vi "ProgramControl-AutoFaultRecovery.vi"(0 "Universal Robot.lvclass in":refnum<class "Universal Robot.lvclass">, 1 "Program":string, 5 "error in (no error)":errorcluster, 9 "Subpanel":refnum<vi>, 11 "Require Normal Mode to Play (F)":bool) -> (14 "Universal Robot.lvclass out":refnum<class "Universal Robot.lvclass">, 15 "programReturnStatus":T1=enum."Complete", 19 "error out":errorcluster)   [LabVIEW 2019, in "Universal Robot.lvclass"]
uses:
  Universal Robot.lvclass
  ProgramReturnStatus.ctl
  ProgramControlFPControls.ctl
  ProgramState.ctl
  SafetyStatus.ctl
  Events/Robot Event/Event Type.ctl
  Events/Robot Event/Robot Event.lvclass
panel:
  out "Loaded Program":string
  out "Message":string
  out "Program Status":string
  in  "Recover":bool
  in  "Resume":bool
  in  "auto fault timeout":i32=1000
  in  "check status timeout":i32=1000
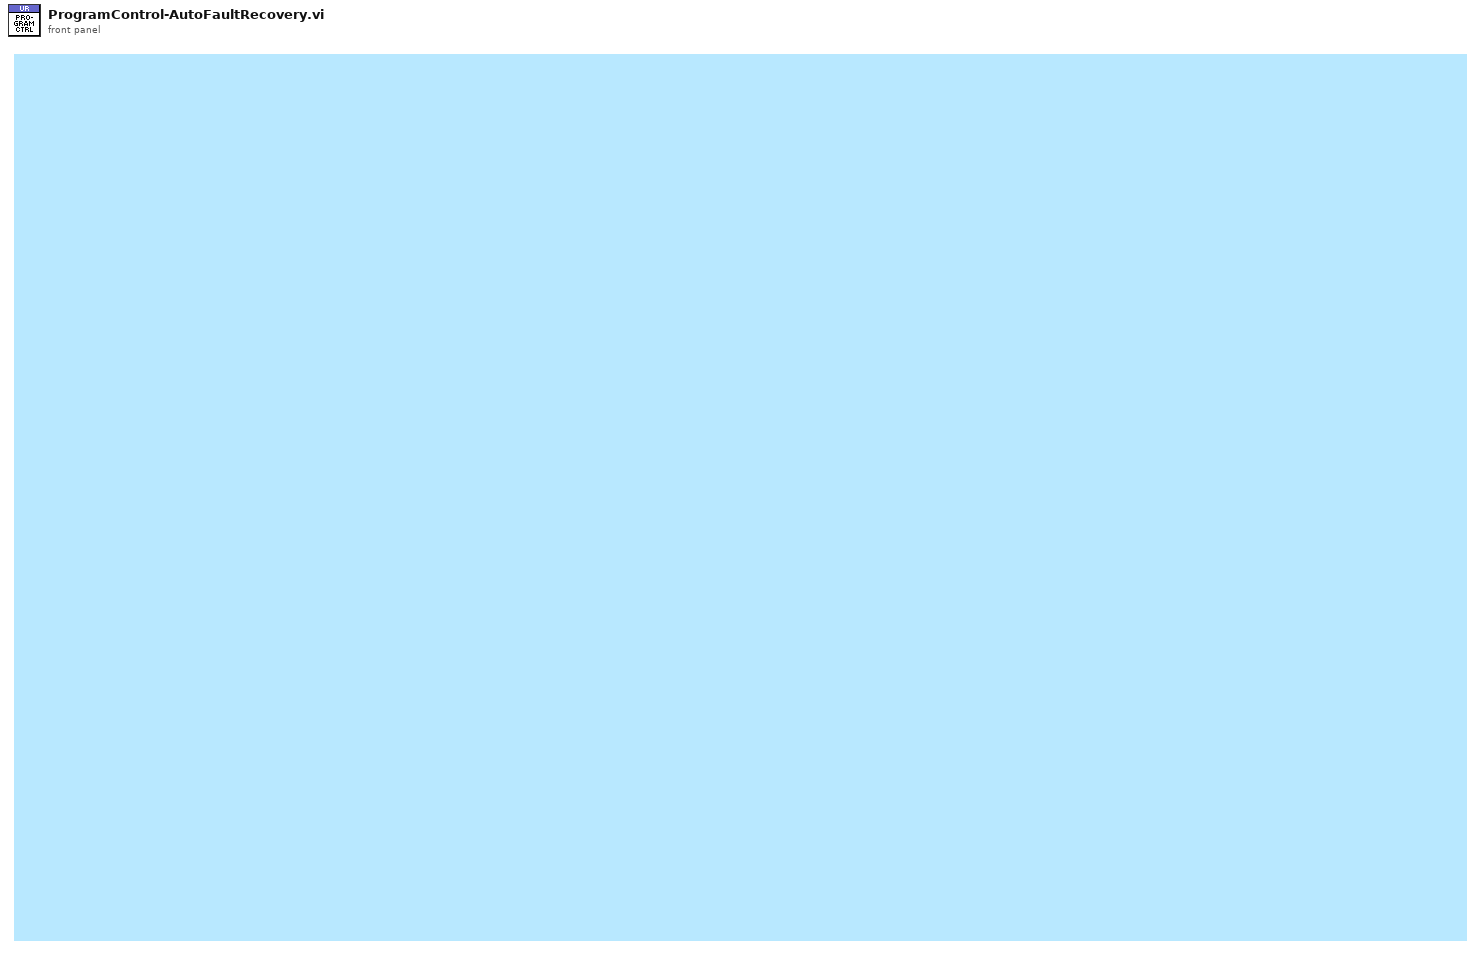
[diagram p1: front panel]
types:
  T1 = typedef "Universal Robot.lvclass/ProgramReturnStatus.ctl" = enum16{"Incomplete", "Complete", "Stopped", "Error", "Faulted", "Timeout"}
  T2 = typedef "Universal Robot.lvclass/ProgramControlFPControls.ctl" = cluster{"Recover Button":refnum<vi>, "Resume Bottom":refnum<vi>, "Message":refnum<vi>, "Program Status":refnum<vi>, "Loaded Program":refnum<vi>, "VI Reference":refnum<vi>, "Time Elapsed":refnum<vi>}
  T3 = typedef "Universal Robot.lvclass/ProgramState.ctl" = enum16{"STOPPED", "PLAYING", "PAUSE"}
  T4 = typedef "Universal Robot.lvclass/SafetyStatus.ctl" = enum16{"INVALID", "NORMAL", "REDUCED", "PROTECTIVE_STOP", "RECOVERY", "SAFEGUARD_STOP", "SYSTEM_EMERGENCY_STOP", "ROBOT_EMERGENCY_STOP", "VIOLATION", "FAULT", "AUTOMATIC_MODE_SAFEGAURD_STOP", "SYSTEM_THREE_POSITION_ENABLING_STOP"}
  T5 = typedef "Robot Event.lvclass/Event Type.ctl" = enum16{"Play", "Error", "Fault", "Timeout", "Fault Auto Recover", "Fault Manual Recover"}
  T6 = enum8{"Enabled", "Disabled", "Disabled and Grayed Out"}
  T7 = typedef "Universal Robot.lvclass/ProgramControlEvent.ctl" = enum16{"Stop", "Pause", "Resume"}
  T8 = typedef "Universal Robot.lvclass/ProgramStatus.ctl" = cluster{"Loaded Program":string, "Valid Program":bool, "Program State":T3, "Running":bool}
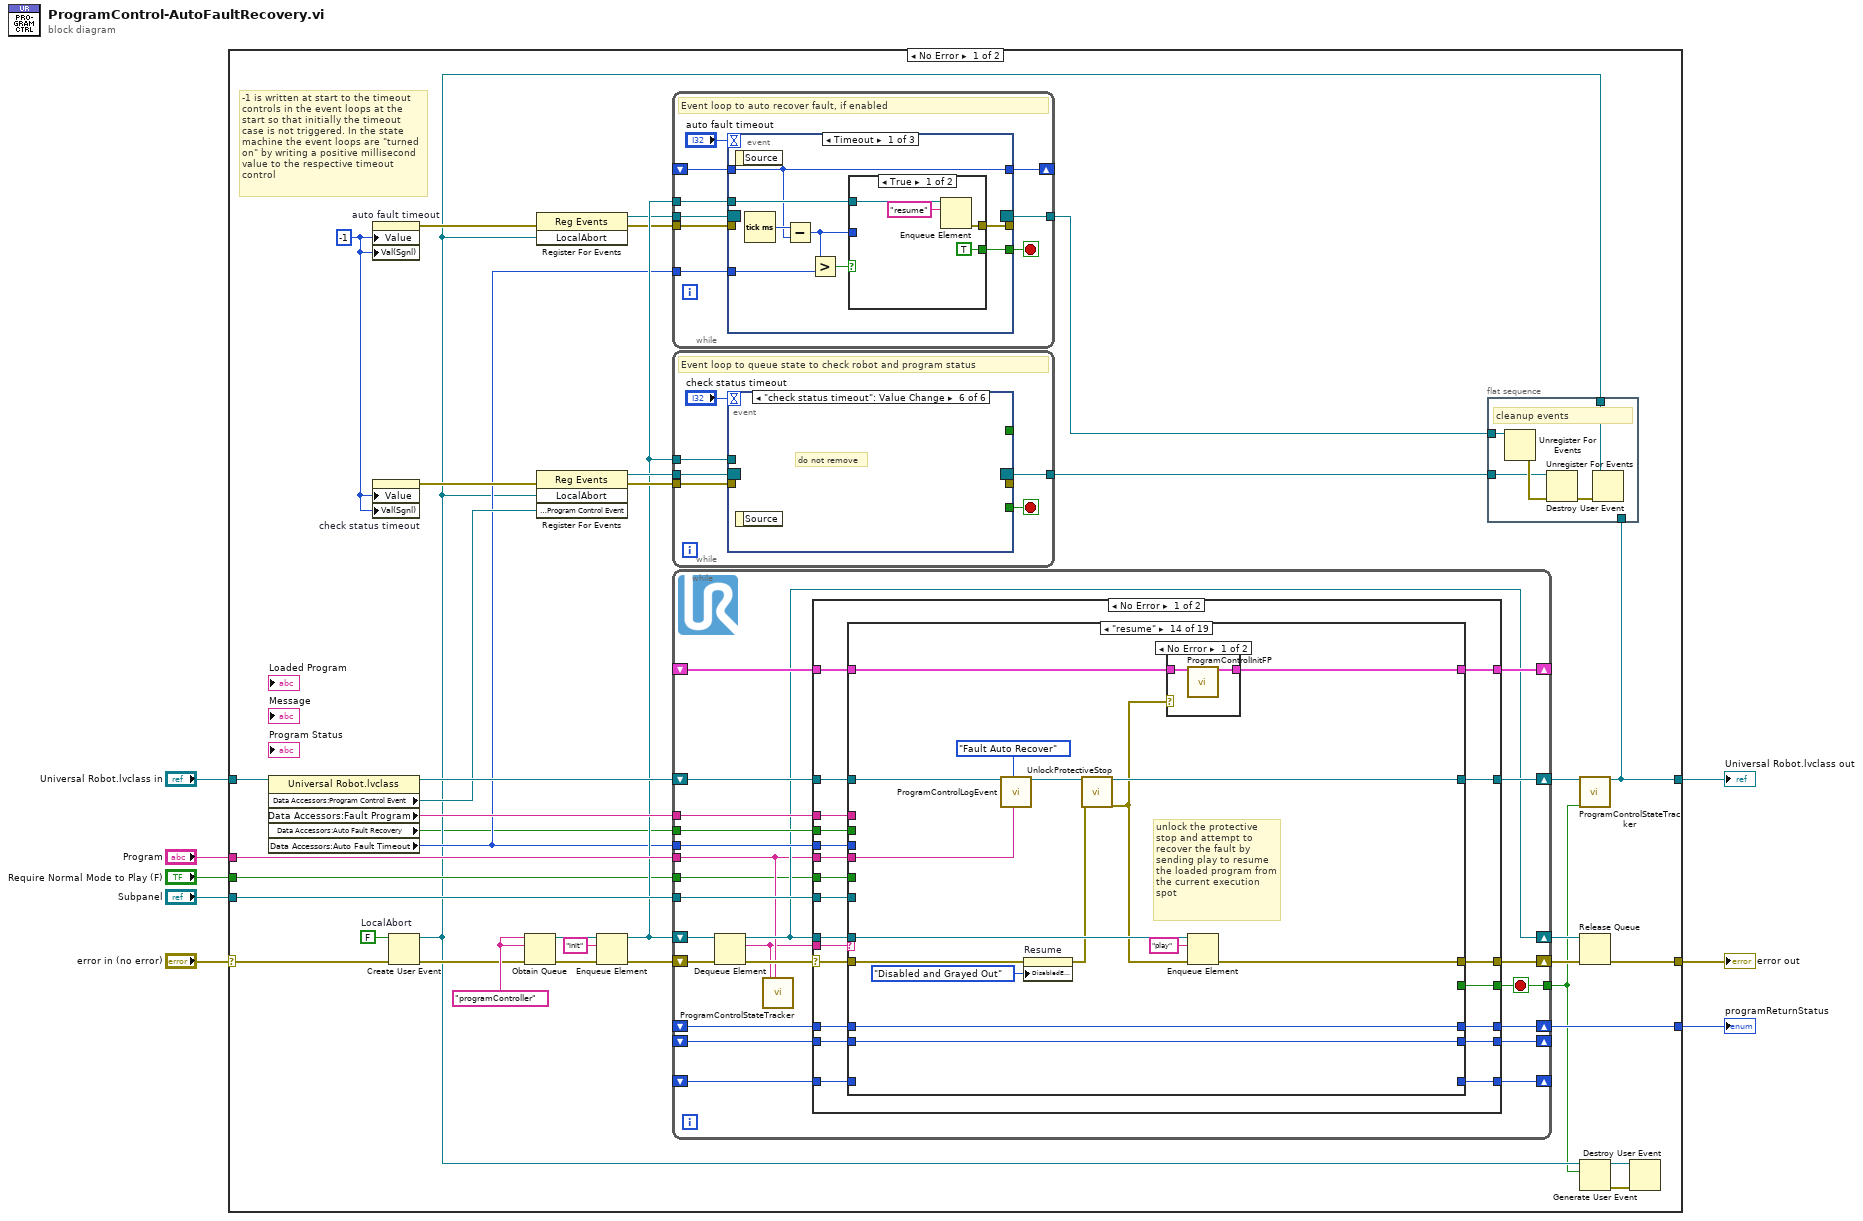
[diagram p0: block diagram]
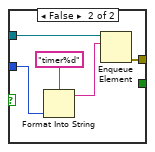
[diagram p2: hidden frame]
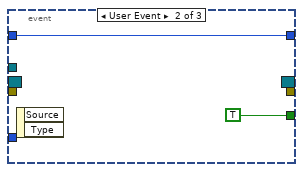
[diagram p3: hidden frame]
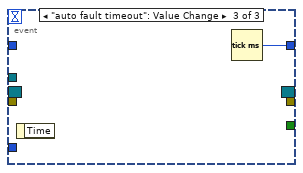
[diagram p4: hidden frame]
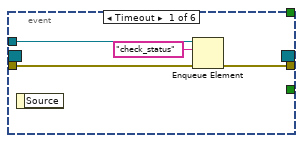
[diagram p5: hidden frame]
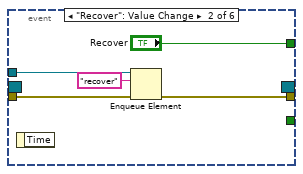
[diagram p6: hidden frame]
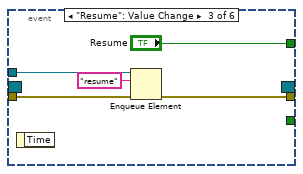
[diagram p7: hidden frame]
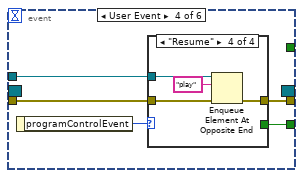
[diagram p8: hidden frame]
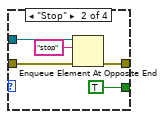
[diagram p10: hidden frame]
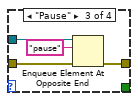
[diagram p11: hidden frame]
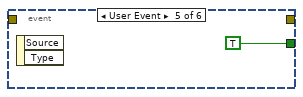
[diagram p12: hidden frame]
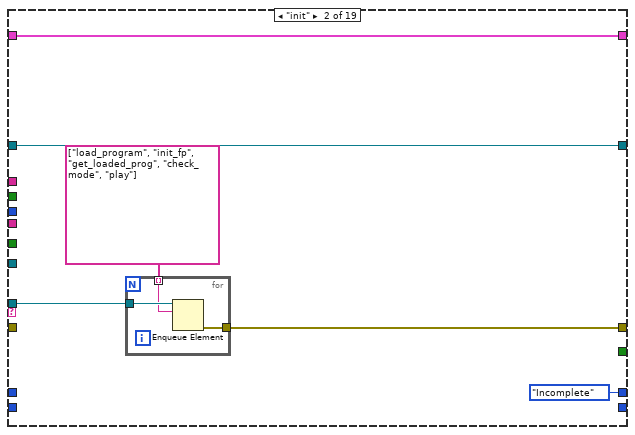
[diagram p14: hidden frame]
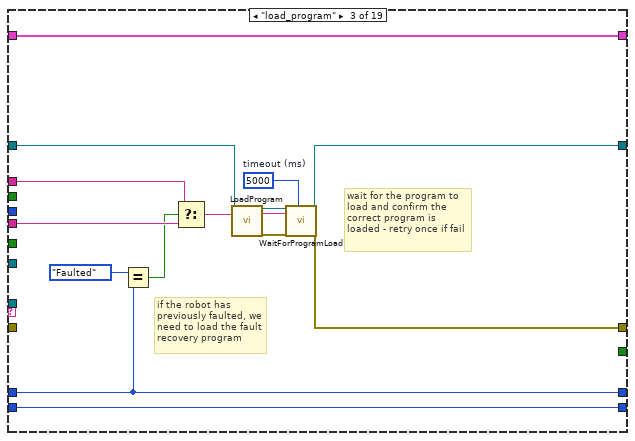
[diagram p15: hidden frame]
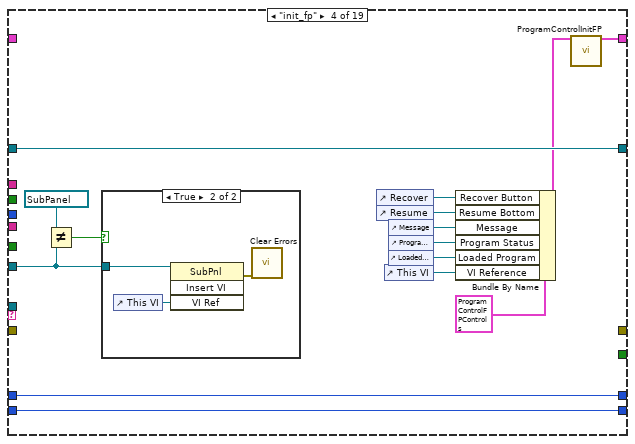
[diagram p16: hidden frame]
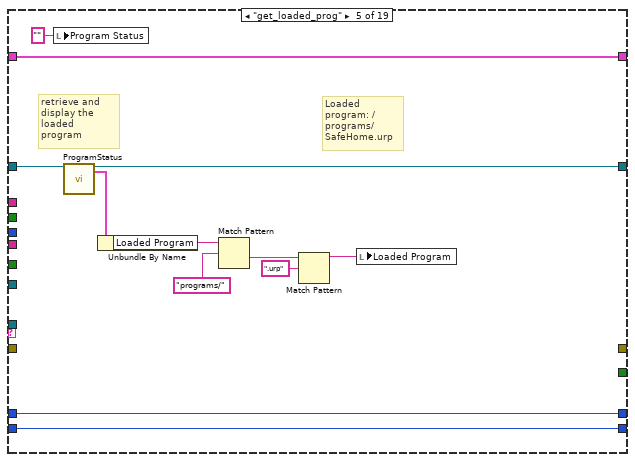
[diagram p18: hidden frame]
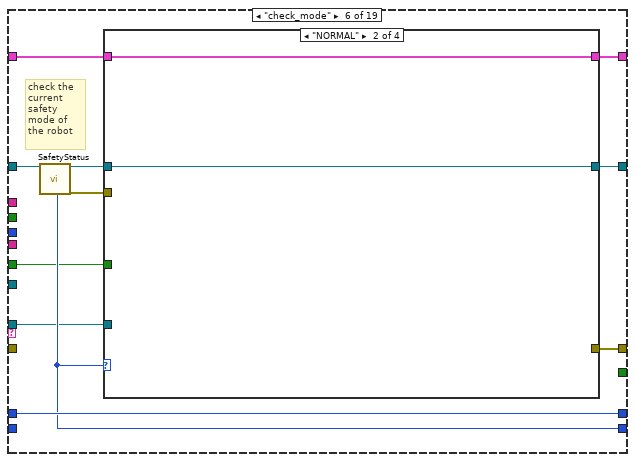
[diagram p19: hidden frame]
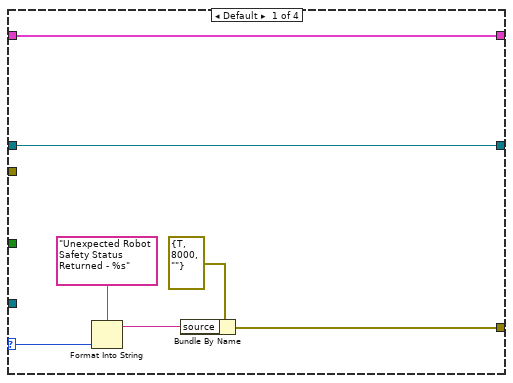
[diagram p20: hidden frame]
diagram:
  n1 = case shown="No Error" "error in (no error)" {
    selector: "error in (no error)" -> [w26 w496]
    tunnel: "Universal Robot.lvclass in" -> [w36 w495]
    tunnel: [w34 _] -> w7
    tunnel: [w27 w496] -> w6
    tunnel: [w11 w495] -> w5
    tunnel: "Subpanel" -> [w25 _]
    tunnel: "Program" -> [w24 _]
    tunnel: "Require Normal Mode to Play (F)" -> [w14 _]
    frame No Error {
      w33 = FALSE  # LocalAbort
      w18 = -1 ("rate")
      w41 = "programController" ("name (unnamed)")
      # "-1 is written at start to the timeout controls in the event loops at the start so that initially the timeout case is not triggered. In the state machine the event loops are \"turned on\" by writing a positive millisecond value to the respective timeout control"
      n2 = property class="Universal Robot.lvclass"(reference=w36) -> (reference out=w40:refnum<class "Universal Robot.lvclass">, "Data Accessors:Program Control Event"=w35:refnum<user-event>, "Data Accessors:Fault Program"=w23:string, "Data Accessors:Auto Fault Recovery"=w10:bool, "Data Accessors:Auto Fault Timeout"=w15:i32)  [unwired: 1 in, 1 out]
      n3 = property on="auto fault timeout" class="DigNum (strict)"("Value"=w18, "Val(Sgnl)"=w18) -> (error out=w19:errorcluster)  [unwired: 2 in, 1 out]
      n4 = property on="check status timeout" class="DigNum (strict)"("Value"=w18, "Val(Sgnl)"=w18) -> (error out=w32:errorcluster)  [unwired: 2 in, 1 out]
      n5 = Create User Event(user event datatype=w33, error in=w26) -> (user event=w12:refnum<user-event>, error out=w31:errorcluster)
      n6 = Obtain Queue(name (unnamed)=w41, element data type=w41, error in (no error)=w31) -> (queue out=w39:refnum<queue>, error out=w38:errorcluster)  [unwired: 2 in, 1 out]
      n7 = register-events(error in=w19, w12) -> (reference out=w20:refnum<event-registration>, error out=w21:errorcluster)  [unwired: 1 in]
      n8 = register-events(error in=w32, w12, w35) -> (reference out=w45:refnum<event-registration>, error out=w44:errorcluster)  [unwired: 1 in]
      n9 = Enqueue Element(queue=w39, element="init", error in (no error)=w38) -> (queue out=w22:refnum<queue>, error out=w37:errorcluster)  [unwired: 1 in, 1 out]
      n10 = while {
        tunnel: w22 -> [w59]
        tunnel: w21 -> [w58]
        tunnel: w20 -> [w57]
        tunnel: [w56] -> w17
        tunnel: w15 -> [w54]
        shift-right: [w53] -> _
        shift-left: _ -> [w52]
        stop <- w51 stop-if-true
        # "Event loop to auto recover fault, if enabled"
        n11 = event shown="[0] Timeout" {
          selector: w57 -> [_ _ _]
          dyn-events: [_ _ _] -> w56
          timeout: "auto fault timeout" -> [_ _ _]
          tunnel: w59 -> [w67 _ _]
          tunnel: w58 -> [_ _ _]
          tunnel: [w66 _ _] -> _
          tunnel: [w60 TRUE _] -> w51
          tunnel: w54 -> [w63 _ _]
          tunnel: [w64 w77 w79] -> w53
          tunnel: w52 -> [w64 w77 _]
          event Timeout {
            n12 = event-data() -> ()  [unwired: 1 in, 1 out]
            n13 = Tick Count (ms)() -> (millisecond timer value=w65:u32)
            n14 = Subtract(x=w65, y=w64) -> (x-y=w61:u32)
            n15 = Greater?(x=w61, y=w63) -> (0:w62:bool)
            n16 = case shown="True" w62 {
              tunnel: w67 -> [w71 w76]
              tunnel: [w70 w75] -> w66
              tunnel: w61 -> [_ w72]
              tunnel: [TRUE _] -> w60
              frame True {
                n17 = Enqueue Element(queue=w71, element="resume") -> (error out=w70:errorcluster)  [unwired: 2 in, 2 out]
              }
              frame False {
                n18 = Format Into String(format string="timer%d" ("element"), w72) -> (resulting string=w73:string)  [unwired: 2 in, 1 out]
                n19 = Enqueue Element(queue=w76, element=w73) -> (error out=w75:errorcluster)  [unwired: 2 in, 2 out]
              }
            }
          }
          event User Event {
            n20 = event-data() -> ()  [unwired: 1 in, 2 out]
          }
          event "auto fault timeout": Value Change {
            n21 = event-data() -> ()  [unwired: 1 in, 1 out]
            n22 = Tick Count (ms)() -> (millisecond timer value=w79:u32)
          }
        }
      }
      n23 = while {
        tunnel: w22 -> [w85]
        tunnel: w44 -> [w84]
        tunnel: w45 -> [w83]
        tunnel: [w81] -> w13
        stop <- w80 stop-if-true
        # "Event loop to queue state to check robot and program status"
        n24 = event shown="[5] \"check status timeout\": Value Change" {
          selector: w83 -> [_ _ _ _ _ _]
          dyn-events: [_ _ _ _ _ _] -> w81
          timeout: "check status timeout" -> [_ _ _ _ _ _]
          tunnel: w85 -> [w89 w94 w99 w104 _ _]
          tunnel: w84 -> [w88 w93 w98 w103 _ _]
          tunnel: [w87 w92 w97 w102 _ _] -> _
          tunnel: [_ _ _ w100 TRUE _] -> w80
          tunnel: [_ "Recover" "Resume" _ _ _] -> _
          event Timeout {
            n25 = event-data() -> ()  [unwired: 1 in, 1 out]
            n26 = Enqueue Element(queue=w89, element="check_status", error in (no error)=w88) -> (error out=w87:errorcluster)  [unwired: 1 in, 2 out]
          }
          event "Recover": Value Change {
            n27 = event-data() -> ()  [unwired: 1 in, 1 out]
            n28 = Enqueue Element(queue=w94, element="recover", error in (no error)=w93) -> (error out=w92:errorcluster)  [unwired: 1 in, 2 out]
          }
          event "Resume": Value Change {
            n29 = event-data() -> ()  [unwired: 1 in, 1 out]
            n30 = Enqueue Element(queue=w99, element="resume", error in (no error)=w98) -> (error out=w97:errorcluster)  [unwired: 1 in, 2 out]
          }
          event User Event {
            n31 = event-data() -> ("programControlEvent"=w101:T7)  [unwired: 1 in]
            n32 = case shown="\"Resume\"" w101 {
              tunnel: w104 -> [_ w110 w114 w118]
              tunnel: w103 -> [w105 w109 w113 w117]
              tunnel: [w105 w108 w112 w116] -> w102
              tunnel: [_ TRUE _ _] -> w100
              frame Default {
              }
              frame "Stop" {
                n33 = Enqueue Element At Opposite End(queue=w110, element="stop", error in (no error)=w109) -> (error out=w108:errorcluster)  [unwired: 1 in, 2 out]
              }
              frame "Pause" {
                n34 = Enqueue Element At Opposite End(queue=w114, element="pause", error in (no error)=w113) -> (error out=w112:errorcluster)  [unwired: 1 in, 2 out]
              }
              frame "Resume" {
                n35 = Enqueue Element At Opposite End(queue=w118, element="play", error in (no error)=w117) -> (error out=w116:errorcluster)  [unwired: 1 in, 2 out]
              }
            }
          }
          event User Event {
            n36 = event-data() -> ()  [unwired: 1 in, 2 out]
          }
          event "check status timeout": Value Change {
            # "do not remove"
            n37 = event-data() -> ()  [unwired: 1 in, 1 out]
          }
        }
      }
      n38 = while {
        shift-right: [w142] -> w43
        shift-left: w37 -> [w127]
        shift-right: [w126] -> w42
        shift-left: w22 -> [w128]
        shift-right: [w140] -> w16
        shift-left: w40 -> [w141]
        tunnel: [w138] -> w9
        tunnel: w25 -> [w137]
        shift-right: [w136] -> _
        shift-left: _ -> [w135]
        tunnel: w24 -> [w124]
        tunnel: w23 -> [w134]
        shift-right: [w139] -> w34
        shift-left: _ -> [w133]
        tunnel: w10 -> [w132]
        shift-right: [w131] -> _
        shift-left: _ -> [w130]
        tunnel: w15 -> [w129]
        tunnel: w14 -> [w123]
        shift-right: [w121] -> _
        shift-left: _ -> [w120]
        stop <- w138 stop-if-true
        n39 = Dequeue Element(queue=w128, error in (no error)=w127) -> (queue out=w126:refnum<queue>, element=w122:string, error out=w125:errorcluster)  [unwired: 1 in, 1 out]
        n40 = call "ProgramControlStateTracker.vi"("State in"=w122, "Program"=w124) -> ()  [unwired: 17 in, 1 out]
        n41 = case shown="No Error" w125 {
          selector: w125 -> [w147 w489]
          tunnel: w126 -> [w148 _]
          tunnel: [w163 w489] -> w142
          tunnel: [w162 TRUE] -> w138
          tunnel: w141 -> [w161 w486]
          tunnel: [w160 w484] -> w140
          tunnel: [w159 ProgramReturnStatus."Error" ("programReturnStatus")] -> w139
          tunnel: w137 -> [w158 _]
          tunnel: [w157 w492] -> w136
          tunnel: w135 -> [w156 w492]
          tunnel: w124 -> [w153 w483]
          tunnel: w134 -> [w155 _]
          tunnel: w133 -> [w154 _]
          tunnel: w132 -> [w152 _]
          tunnel: [w151 w491] -> w131
          tunnel: w130 -> [w150 w491]
          tunnel: w129 -> [w149 _]
          tunnel: w122 -> [w146 _]
          tunnel: w123 -> [w145 _]
          tunnel: [w144 _] -> w121
          tunnel: w120 -> [w143 _]
          frame No Error {
            n42 = case shown="\"resume\"" w146 {
              selector: w146 -> [_ _ _ _ _ _ _ _ _ _ _ _ w405 _ _ _ _ _ _]
              tunnel: w147 -> [w168 _ _ _ _ _ _ _ _ _ _ w376 _ w412 w432 _ _ _ _]
              tunnel: w148 -> [_ w172 _ _ _ w230 w277 _ _ w320 w360 w387 _ w423 w441 _ _ _ _]
              tunnel: [w168 w171 w182 _ _ w231 w278 errorcluster {"status"=TRUE, "code"=8000, "source"="Timed out waiting for program to play"} ("error out") _ w319 _ _ _ w409 w429 w454 w463 w473 _] -> w163
              tunnel: [_ _ _ _ _ _ _ TRUE _ _ w357 _ _ _ _ TRUE TRUE _ TRUE] -> w162
              tunnel: w161 -> [w167 w174 w191 w198 w222 w228 w282 w301 w306 w312 w362 w385 w407 w416 w436 w456 w465 w477 w481]
              tunnel: [w167 w174 w183 w198 w221 w226 w270 w301 w306 w318 w362 w384 w407 w414 w440 w455 w464 w474 w481] -> w160
              tunnel: [w165 ProgramReturnStatus."Incomplete" ("programReturnStatus") w187 w199 w214 w233 w272 ProgramReturnStatus."Error" ("programReturnStatus") w303 w314 w358 w386 w406 w419 ProgramReturnStatus."Faulted" ("programReturnStatus") w458 ProgramReturnStatus."Stopped" ("programReturnStatus") w469 ProgramReturnStatus."Error" ("programReturnStatus")] -> w159
              tunnel: w158 -> [_ _ _ w207 _ _ _ _ _ _ _ _ _ _ _ _ _ _ _]
              tunnel: [w166 w173 w192 w200 w213 w223 w265 w298 w304 w317 w361 w388 w401 w420 w444 w457 w460 w471 w480] -> w157
              tunnel: w156 -> [w166 w173 w192 _ w213 w224 w265 w298 w304 w309 w361 w389 w401 w421 w444 w457 w460 w471 w480]
              tunnel: w153 -> [_ _ w190 _ _ _ w268 _ _ _ _ w383 _ w413 w434 _ _ _ _]
              tunnel: w155 -> [_ _ w189 _ _ _ _ _ _ _ _ _ _ _ _ _ _ _ _]
              tunnel: w154 -> [w165 _ w187 w199 w214 w233 w272 _ w303 w315 w359 w386 w406 w419 _ w458 _ w469 _]
              tunnel: w152 -> [_ _ _ _ _ _ _ _ _ _ _ w381 _ _ _ _ _ _ _]
              tunnel: [w164 _ w184 w195 w212 w232 w267 w296 w302 w316 w355 w380 w397 w418 w437 w452 w459 w468 w478] -> w151
              tunnel: w150 -> [w164 _ w184 w195 w212 _ w267 w296 w302 w313 w356 w380 w397 w418 w437 w452 w459 w468 w478]
              tunnel: w149 -> [_ _ _ _ _ _ _ _ _ _ _ _ w396 _ _ _ _ _ _]
              tunnel: w145 -> [_ _ _ _ _ w225 _ _ _ _ _ _ _ _ _ _ _ _ _]
              tunnel: [_ _ _ _ _ _ _ _ _ w307 w354 w374 _ _ _ _ _ _ _] -> w144
              tunnel: w143 -> [_ _ _ _ _ _ _ _ _ _ w354 w374 _ _ _ _ _ _ _]
              frame Default {
              }
              frame "init" {
                n43 = for {
                  tunnel: w172 -> [w177]
                  tunnel: [w176] -> w171
                  tunnel: string[] ["load_program", "init_fp", "get_loaded_prog", "check_mode", "play"] -> [w175] mode=indexing
                  n44 = Enqueue Element(queue=w177, element=w175) -> (error out=w176:errorcluster)  [unwired: 2 in, 2 out]
                }
              }
              frame "load_program" {
                w178 = u32 5000  # timeout (ms)
                # "wait for the program to load and confirm the correct program is loaded - retry once if fail"
                # "if the robot has previously faulted, we need to load the fault recovery program"
                n45 = Equal?(x=ProgramReturnStatus."Faulted", y=w187) -> (x = y?=w185:bool)
                n46 = Select(t=w189, s=w185, f=w190) -> (s? t:f=w188:string)
                n47 = call-dynamic "LoadProgram.vi"("Universal Robot.lvclass in"=w191, "program in"=w188) -> ("Universal Robot.lvclass out"=w180:refnum<class "Universal Robot.lvclass">, "program out"=w179:string, "error out"=w181:errorcluster)  [unwired: 15 in]
                n48 = call-dynamic "WaitForProgramLoad.vi"("Universal Robot.lvclass in"=w180, "program in"=w179, "error in (no error)"=w181, "timeout (ms)"=w178) -> ("Universal Robot.lvclass out"=w183:refnum<class "Universal Robot.lvclass">, "error out"=w182:errorcluster)  [unwired: 14 in]
              }
              frame "init_fp" {
                n49 = Not Equal?(x=refnum<vi> refnum, y=w207) -> (x != y?=w205:bool)
                n50 = case shown="True" w205 {
                  tunnel: w207 -> [_ w210]
                  frame False {
                  }
                  frame True {
                    n51 = control-ref of="This VI"() -> (w208:refnum<vi>)
                    n52 = invoke class="SubPnl" method="Insert VI"(reference=w210, "VI Ref"=w208) -> (error out=w209:errorcluster)  [unwired: 2 in, 3 out]
                    n53 = call <vilib>:"Clear Errors.vi"("error in (no error)"=w209) -> ()  [unwired: 5 in, 2 out]
                  }
                }
                n54 = control-ref of="Recover"() -> (w204:refnum<vi>)
                n55 = control-ref of="Resume"() -> (w203:refnum<vi>)
                n56 = control-ref of="This VI"() -> (w193:refnum<vi>)
                n57 = control-ref of="Message"() -> (w202:refnum<vi>)
                n58 = control-ref of="Program Status"() -> (w201:refnum<vi>)
                n59 = control-ref of="Loaded Program"() -> (w194:refnum<vi>)
                n60 = Bundle By Name(cluster=T2 {"Recover Button"=refnum, "Resume Bottom"=refnum, "Message"=refnum, "Program Status"=refnum, "Loaded Program"=refnum, "VI Reference"=refnum, "Time Elapsed"=refnum} ("Front Panel Controls"), "Recover Button"=w204, "Resume Bottom"=w203, "Message"=w202, "Program Status"=w201, "Loaded Program"=w194, "VI Reference"=w193) -> (w196:T2)
                n61 = call "ProgramControlInitFP.vi"("Front Panel Controls in"=w196) -> ("Front Panel Controls out"=w200:T2)  [unwired: 18 in]
              }
              frame "get_loaded_prog" {
                # "Loaded program: /programs/SafeHome.urp"
                # "retrieve and display the loaded program"
                n62 = local write "Program Status"("" ("Program Status")) -> ()
                n63 = call-dynamic "ProgramStatus.vi"("Universal Robot.lvclass in"=w222) -> ("Universal Robot.lvclass out"=w221:refnum<class "Universal Robot.lvclass">, "Program Status"=w220:T8)  [unwired: 16 in, 1 out]
                n64 = Unbundle By Name(w220) -> ("Loaded Program"=w218:string)
                n65 = Match Pattern(string=w218, regular expression="programs/") -> (after substring=w216:string)  [unwired: 1 in, 3 out]
                n66 = Match Pattern(string=w216, regular expression=".urp") -> (before substring=w211:string)  [unwired: 1 in, 3 out]
                n67 = local write "Loaded Program"(w211) -> ()
              }
              frame "check_mode" {
                # "check the current safety mode of the robot"
                n68 = call-dynamic "SafetyStatus.vi"("Universal Robot.lvclass in"=w228) -> ("safetyStatus out"=w232:T4, "Universal Robot.lvclass out"=w227:refnum<class "Universal Robot.lvclass">, "error out"=w229:errorcluster)  [unwired: 16 in]
                n69 = case shown="\"NORMAL\"" w232 {
                  selector: w232 -> [w236 _ _ _]
                  tunnel: w229 -> [_ _ _ _]
                  tunnel: [w237 _ w247 w263] -> w231
                  tunnel: w230 -> [_ _ w248 w264]
                  tunnel: w227 -> [w235 w242 w245 w261]
                  tunnel: [w235 w242 w246 w261] -> w226
                  tunnel: w225 -> [_ _ w244 _]
                  tunnel: w224 -> [w234 w241 w243 w260]
                  tunnel: [w234 w241 w243 w260] -> w223
                  frame Default {
                    n70 = Format Into String(format string="Unexpected Robot Safety Status Returned - %s", w236) -> (resulting string=w240:string)  [unwired: 2 in, 1 out]
                    n71 = Bundle By Name(cluster=errorcluster {"status"=TRUE, "code"=8000, "source"=""} ("error constant"), "source"=w240) -> (w237:errorcluster)
                  }
                  frame "NORMAL" {
                  }
                  frame "REDUCED" {
                    # "check to see if the robot must be in normal mode to begin playing the loaded program"
                    n72 = case shown="True" w244 {
                      tunnel: w248 -> [_ w259]
                      tunnel: [_ w258] -> w247
                      tunnel: w245 -> [w249 w254]
                      tunnel: [w249 w254] -> w246
                      tunnel: w243 -> [_ w252]
                      frame False {
                      }
                      frame True {
                        # "enqueue same state at front to loop back and continue checking"
                        n73 = Unbundle By Name(w252) -> ("Program Status"=w251:refnum<vi>, "Message"=w255:refnum<vi>)
                        n74 = property class="Str"(reference=w255, "Value"="Robot must be in Normal Mode to Start Program\n\nPlease Vacate any Active Protection Zones to Continue" ("element")) -> ()  [unwired: 1 in, 2 out]
                        n75 = Wait (ms)(milliseconds to wait=u32 500) -> ()  [unwired: 1 out]
                        n76 = Enqueue Element At Opposite End(queue=w259, element="check_mode") -> (error out=w258:errorcluster)  [unwired: 2 in, 2 out]
                        n77 = property class="Str"(reference=w251, "Value"="REDUCED MODE" ("element")) -> ()  [unwired: 1 in, 2 out]
                      }
                    }
                  }
                  frame "PROTECTIVE_STOP" {
                    # "program cannot be played because a protective stop is on - move to fault case"
                    n78 = Enqueue Element At Opposite End(queue=w264, element="fault") -> (error out=w263:errorcluster)  [unwired: 2 in, 2 out]
                  }
                }
              }
              frame "play" {
                # "play the program and wait  until it begins playing or a timeout is reached"
                n79 = call-dynamic "Play.vi"("Universal Robot.lvclass in"=w282) -> ("Universal Robot.lvclass out"=w281:refnum<class "Universal Robot.lvclass">, "error out"=w280:errorcluster)  [unwired: 17 in]
                n80 = Tick Count (ms)() -> (millisecond timer value=w279:u32)
                n81 = while {
                  shift-right: [w284] -> w271
                  shift-left: w281 -> [w287]
                  tunnel: w280 -> [w286]
                  tunnel: w279 -> [w294]
                  tunnel: [w285] -> w266
                  tunnel: [w292] -> w276
                  tunnel: [w288] -> w269
                  stop <- w289 stop-if-true
                  # "Wait for program to start"
                  n82 = call-dynamic "ProgramState.vi"("Universal Robot.lvclass in"=w287, "error in (no error)"=w286) -> ("Universal Robot.lvclass out"=w284:refnum<class "Universal Robot.lvclass">, "programState out"=w283:T3, "error out"=w285:errorcluster)  [unwired: 15 in]
                  n83 = Tick Count (ms)() -> (millisecond timer value=w295:u32)
                  n84 = Subtract(x=w295, y=w294) -> (x-y=w288:u32)
                  n85 = Greater?(x=w288, y=u32 5000) -> (0:w292:bool)
                  n86 = Equal?(x=ProgramState."PLAYING", y=w283) -> (x = y?=w290:bool)
                  n87 = Or(x=w290, y=w292) -> (x .or. y?=w289:bool)
                }
                n88 = Select(t="startup_error", s=w276, f="start_program_control") -> (s? t:f=w274:string)
                n89 = Enqueue Element(queue=w277, element=w274, error in (no error)=w266) -> (error out=w278:errorcluster)  [unwired: 1 in, 2 out]
                n90 = call "ProgramControlLogEvent.vi"("Universal Robot.lvclass"=w271, "data"=w269, "Program"=w268) -> ("Universal Robot.lvclass out"=w270:refnum<class "Universal Robot.lvclass">)  [unwired: 16 in]
              }
              frame "startup_error" {
                # "the application timed out waiting for the loaded program to start\n\ncheck the teach pendant for errors"
              }
              frame "start_program_control" {
                w305 = 500 ("rate")
                # "turn on timeout event which is used to check program status"
                n91 = property on="check status timeout" class="DigNum (strict)"("Value"=w305, "Val(Sgnl)"=w305) -> ()  [unwired: 2 in, 2 out]
              }
              frame "check_status" {
                (unwired) SafetyStatus."INVALID"  # Safety Status
                # "check the robot safety status"
                n92 = call-dynamic "SafetyStatus.vi"("Universal Robot.lvclass in"=w312) -> ("safetyStatus out"=w307:T4, "Universal Robot.lvclass out"=w311:refnum<class "Universal Robot.lvclass">, "error out"=w310:errorcluster)  [unwired: 16 in]
                n93 = call "ProgramControlSafetyMode.vi"("Front Panel Controls in"=w309, "Safety Status"=w307) -> ("Front Panel Controls out"=w308:T2)  [unwired: 17 in]
                n94 = case shown="\"NORMAL\", \"REDUCED\"" w307 {
                  selector: w307 -> [w327 _ w348]
                  tunnel: w320 -> [w332 w341 _]
                  tunnel: [w331 w342 w346] -> w319
                  tunnel: [w322 w344 w353] -> w318
                  tunnel: w311 -> [w325 w344 w353]
                  tunnel: w310 -> [w324 _ _]
                  tunnel: w308 -> [w330 w340 w352]
                  tunnel: [w330 w340 w352] -> w317
                  tunnel: [w327 w339 w351] -> w316
                  tunnel: w315 -> [w326 w338 w350]
                  tunnel: [w326 w338 w350] -> w314
                  tunnel: w313 -> [_ w339 w351]
                  frame "NORMAL", "REDUCED" {
                    # "determine if the program has completed"
                    n95 = call-dynamic "ProgramState.vi"("Universal Robot.lvclass in"=w325, "error in (no error)"=w324) -> ("Universal Robot.lvclass out"=w322:refnum<class "Universal Robot.lvclass">, "programState out"=w321:T3, "error out"=w323:errorcluster)  [unwired: 15 in]
                    n96 = Unbundle By Name(w330) -> ("Program Status"=w329:refnum<vi>)
                    n97 = Format Into String(w321) -> (resulting string=w328:string)  [unwired: 3 in, 1 out]
                    n98 = case shown="\"STOPPED\"" w321 {
                      tunnel: w332 -> [w336 _]
                      tunnel: w323 -> [w335 w337]
                      tunnel: [w334 w337] -> w331
                      frame "STOPPED" {
                        n99 = Enqueue Element At Opposite End(queue=w336, element="program_ended", error in (no error)=w335) -> (error out=w334:errorcluster)  [unwired: 1 in, 2 out]
                      }
                      frame Default {
                      }
                    }
                    n100 = property class="Str"(reference=w329, "Value"=w328) -> ()  [unwired: 1 in, 2 out]
                  }
                  frame "PROTECTIVE_STOP" {
                    # "protective stop was triggered, alert the user"
                    n101 = Enqueue Element At Opposite End(queue=w341, element="fault") -> (error out=w342:errorcluster)  [unwired: 2 in, 2 out]
                  }
                  frame Default {
                    # "an unhandled safety status was returned, need to create an error"
                    n102 = Format Into String(format string="Unexpected Robot Safety Status Returned - %s", w348) -> (resulting string=w345:string)  [unwired: 2 in, 1 out]
                    n103 = Bundle By Name(cluster=errorcluster {"status"=TRUE, "code"=8000, "source"=""} ("error constant"), "source"=w345) -> (w346:errorcluster)
                  }
                }
              }
              frame "program_ended" {
                n104 = case shown="\"Faulted\"" w359 {
                  selector: w359 -> [_ w367]
                  tunnel: w360 -> [_ w368]
                  tunnel: [ProgramReturnStatus."Complete" ("programReturnStatus") w367] -> w358
                  tunnel: [TRUE _] -> w357
                  tunnel: w356 -> [w363 w366]
                  tunnel: [w363 w366] -> w355
                  frame "Complete", Default {
                  }
                  frame "Faulted" {
                    n105 = for {
                      tunnel: w368 -> [w372]
                      tunnel: [w371] -> _
                      tunnel: string[] ["manual_recover"] -> [w370] mode=indexing
                      n106 = Enqueue Element(queue=w372, element=w370) -> (error out=w371:errorcluster)  [unwired: 2 in, 2 out]
                    }
                  }
                }
              }
              frame "fault" {
                w390 = -1 ("rate")
                # "flush queue to prevent strange behavior"
                # "for auto fault recovery to be available, the robot must have been running in normal mode prior to fault - if it was in reduced mode auto fault is not available"
                # "check status event loop is temporarily disabled"
                # "if auto fault recovery is enabled, start a timeout event case using the auto fault timeout value\n\nafter the timeout has elapsed, the fault will auto recover\n\nthis can only be done once!"
                # "make fault recovery buttons visible"
                n107 = Format Into String(w374) -> (resulting string=w373:string)  [unwired: 3 in, 1 out]
                n108 = property on="check status timeout" class="DigNum (strict)"(error in=w376, "Value"=w390, "Val(Sgnl)"=w390) -> (error out=w375:errorcluster)  [unwired: 1 in, 1 out]
                n109 = call "ProgramControlFault.vi"("Front Panel Controls in"=w389) -> ("Front Panel Controls out"=w388:T2)  [unwired: 18 in]
                n110 = call "ProgramControlLogEvent.vi"("Universal Robot.lvclass"=w385, "data"=w373, "Event Type"=Event_Type."Fault", "Program"=w383) -> ("Universal Robot.lvclass out"=w384:refnum<class "Universal Robot.lvclass">)  [unwired: 15 in]
                n111 = Flush Queue(queue=w387, error in (no error)=w375) -> ()  [unwired: 3 out]
                n112 = Equal?(x=SafetyStatus."NORMAL", y=w380) -> (x = y?=w378:bool)
                n113 = And(x=w381, y=w378) -> (x .and. y?=w377:bool)
                n114 = case shown="True" w377 {
                  frame False {
                  }
                  frame True {
                    w391 = 250 ("auto fault timeout")
                    n115 = property on="auto fault timeout" class="DigNum (strict)"("Value"=w391, "Val(Sgnl)"=w391) -> ()  [unwired: 2 in, 2 out]
                  }
                }
              }
              frame "timer".."timer~" {
                n116 = Match Pattern(string=w405, regular expression="timer") -> (after substring=w403:string)  [unwired: 1 in, 3 out]
                n117 = Decimal String To Number(string=w403) -> (number=w395:i32)  [unwired: 2 in, 1 out]
                n118 = Subtract(x=w396, y=w395) -> (x-y=w394:i32)
                n119 = Unbundle By Name(w401) -> ("Program Status"=w402:refnum<vi>)
                n120 = Divide(x=w394, y=1000) -> (x/y=w393:dbl)
                n121 = Format Into String(format string="AUTO RECOVERING FAULT IN %.2f SECONDS", w393) -> (resulting string=w398:string)  [unwired: 2 in, 1 out]
                n122 = property class="Str"(reference=w402, "Text.FontSize"=u32 48 ("Text.Font:Size"), "Value"=w398) -> ()  [unwired: 1 in, 2 out]
              }
              frame "resume" {
                # "unlock the protective stop and attempt to recover the fault by sending play to resume the loaded program from the current execution spot"
                n123 = call "ProgramControlLogEvent.vi"("Universal Robot.lvclass"=w416, "Event Type"=Event_Type."Fault Auto Recover", "Program"=w413) -> ("Universal Robot.lvclass out"=w415:refnum<class "Universal Robot.lvclass">)  [unwired: 16 in]
                n124 = property on="Resume" class="Bool"(error in=w412, "DisabledEnum"=T6."Disabled and Grayed Out" ("Disabled")) -> (error out=w410:errorcluster)  [unwired: 1 in, 1 out]
                n125 = call-dynamic "UnlockProtectiveStop.vi"("Universal Robot.lvclass in"=w415, "error in (no error)"=w410) -> ("Universal Robot.lvclass out"=w414:refnum<class "Universal Robot.lvclass">, "error out"=w408:errorcluster)  [unwired: 16 in]
                n126 = case shown="No Error" w408 {
                  tunnel: w421 -> [w425 w426]
                  tunnel: [w424 w426] -> w420
                  frame No Error {
                    n127 = call "ProgramControlInitFP.vi"("Front Panel Controls in"=w425) -> ("Front Panel Controls out"=w424:T2)  [unwired: 18 in]
                  }
                  frame Error {
                  }
                }
                n128 = Enqueue Element(queue=w423, element="play", error in (no error)=w408) -> (error out=w409:errorcluster)  [unwired: 1 in, 2 out]
              }
              frame "recover" {
                n129 = call "ProgramControlLogEvent.vi"("Universal Robot.lvclass"=w436, "Event Type"=Event_Type."Fault Manual Recover", "Program"=w434) -> ("Universal Robot.lvclass out"=w435:refnum<class "Universal Robot.lvclass">)  [unwired: 16 in]
                n130 = property on="Recover" class="Bool"(error in=w432, "DisabledEnum"=T6."Disabled and Grayed Out" ("Disabled")) -> (error out=w430:errorcluster)  [unwired: 1 in, 1 out]
                n131 = call-dynamic "UnlockProtectiveStop.vi"("Universal Robot.lvclass in"=w435, "error in (no error)"=w430) -> ("Universal Robot.lvclass out"=w440:refnum<class "Universal Robot.lvclass">, "error out"=w439:errorcluster)  [unwired: 16 in]
                n132 = for {
                  tunnel: w441 -> [w451]
                  tunnel: [w450] -> w438
                  tunnel: string[] ["load_program", "get_loaded_prog", "play"] -> [w449] mode=indexing
                  tunnel: w439 -> [w448]
                  n133 = Enqueue Element(queue=w451, element=w449, error in (no error)=w448) -> (error out=w450:errorcluster)  [unwired: 1 in, 2 out]
                }
                n134 = flat-sequence {
                  tunnel: w438 -> [w446]
                  tunnel: [w446] -> w428
                  tunnel: [T6."Enabled" ("Disabled")] -> w427
                  frame #0 {
                    n135 = Wait (ms)(milliseconds to wait=u32 500) -> ()  [unwired: 1 out]
                  }
                }
                n136 = property on="Recover" class="Bool"(error in=w428, "DisabledEnum"=w427) -> (error out=w429:errorcluster)  [unwired: 1 in, 1 out]
              }
              frame "manual_recover" {
                # "tcp connection is closed by peer after setting auto mode, so reconnection needed"
                n137 = call-dynamic "SetAutomaticMode.vi"("Universal Robot.lvclass in"=w456) -> ("Universal Robot.lvclass out"=w455:refnum<class "Universal Robot.lvclass">, "error out"=w454:errorcluster)  [unwired: 17 in]
              }
              frame "stop" {
                w462 = -1 ("rate")
                n138 = property on="check status timeout" class="DigNum (strict)"("Value"=w462, "Val(Sgnl)"=w462) -> (error out=w461:errorcluster)  [unwired: 2 in, 1 out]
                n139 = call-dynamic "Stop.vi"("Universal Robot.lvclass in"=w465, "error in (no error)"=w461) -> ("Universal Robot.lvclass out"=w464:refnum<class "Universal Robot.lvclass">, "error out"=w463:errorcluster)  [unwired: 16 in]
              }
              frame "pause" {
                w476 = -1 ("rate")
                n140 = property on="check status timeout" class="DigNum (strict)"("Value"=w476, "Val(Sgnl)"=w476) -> (error out=w475:errorcluster)  [unwired: 2 in, 1 out]
                n141 = Unbundle By Name(w471) -> ("Program Status"=w472:refnum<vi>)
                n142 = call-dynamic "Pause.vi"("Universal Robot.lvclass in"=w477, "error in (no error)"=w475) -> ("Universal Robot.lvclass out"=w474:refnum<class "Universal Robot.lvclass">, "error out"=w473:errorcluster)  [unwired: 16 in]
                n143 = property class="Str"(reference=w472, "Value"="PAUSED") -> ()  [unwired: 1 in, 2 out]
              }
              frame "abort" {
              }
            }
          }
          frame Error {
            n144 = Unbundle By Name(w489) -> ("source"=w488:string)
            n145 = call "ProgramControlLogEvent.vi"("Universal Robot.lvclass"=w486, "data"=w488, "Event Type"=Event_Type."Error", "Program"=w483) -> ("Universal Robot.lvclass out"=w485:refnum<class "Universal Robot.lvclass">)  [unwired: 15 in]
            n146 = call "ProgramControlStateTracker.vi"("Universal Robot.lvclass"=w485, "State in"="error", "Program"=w483) -> ("Universal Robot.lvclass out"=w484:refnum<class "Universal Robot.lvclass">)  [unwired: 16 in]
          }
        }
      }
      n147 = flat-sequence {
        tunnel: w17 -> [w50]
        tunnel: w13 -> [w48]
        tunnel: w12 -> [w46]
        tunnel: w11 -> [_]
        frame #0 {
          # "cleanup events"
          n148 = Unregister For Events(event registration refnum=w50) -> (error out=w49:errorcluster)  [unwired: 1 in]
          n149 = Unregister For Events(event registration refnum=w48, error in=w49) -> (error out=w47:errorcluster)
          n150 = Destroy User Event(user event=w46, error in=w47) -> ()  [unwired: 1 out]
        }
      }
      n151 = call "ProgramControlStateTracker.vi"("Universal Robot.lvclass"=w16, "Complete (F)"=w9) -> ("Universal Robot.lvclass out"=w11:refnum<class "Universal Robot.lvclass">)  [unwired: 17 in]
      n152 = Release Queue(queue=w42, error in (no error)=w43) -> (error out=w27:errorcluster)  [unwired: 1 in, 2 out]
      n153 = Generate User Event(user event=w12, event data cluster=w9) -> (user event out=w29:refnum<user-event>, error out=w28:errorcluster)  [unwired: 2 in]
      n154 = Destroy User Event(user event=w29, error in=w28) -> ()  [unwired: 1 out]
    }
    frame Error {
    }
  }
  "error out" <- w6
  "Universal Robot.lvclass out" <- w5
  "programReturnStatus" <- w7
